vi "QTrkFree.vi"(4 "error in (no error)":errorcluster, 7 "QTrk Instance":T1={"QTrk Pointer"=0, "QTrk Settings"={"Image width"=150, "Image height"=150, "Number of threads (CPU based)"=-1, "Max Queue Size"=128, "XCOR Profile Length"=32, "XCOR Profile Width"=2, "XCOR Iterations"=5, "ZLUT MinRadius"=50.0, "ZLUT MaxRadius"=64.0, "ZLUT AngularSteps"=0, "QI Iterations"=64, "QI RadialSteps"=64, "QI AngularSteps Per Quadrant"=2, "QI MinRadius"=50.0, "QI MaxRadius"=50.0, "CUDA Device# (if using cuda)"=0, "COM Background correction factor"=2.0, "ZLUT RadialSteps"=32, "Gaussian 2D Fit Iterations"=8}}) -> (0 "error out":errorcluster)   [LabVIEW 2011]
uses:
  QTrkInstance.ctl
  QTrkSettings.ctl
  QTrkDLL.vi
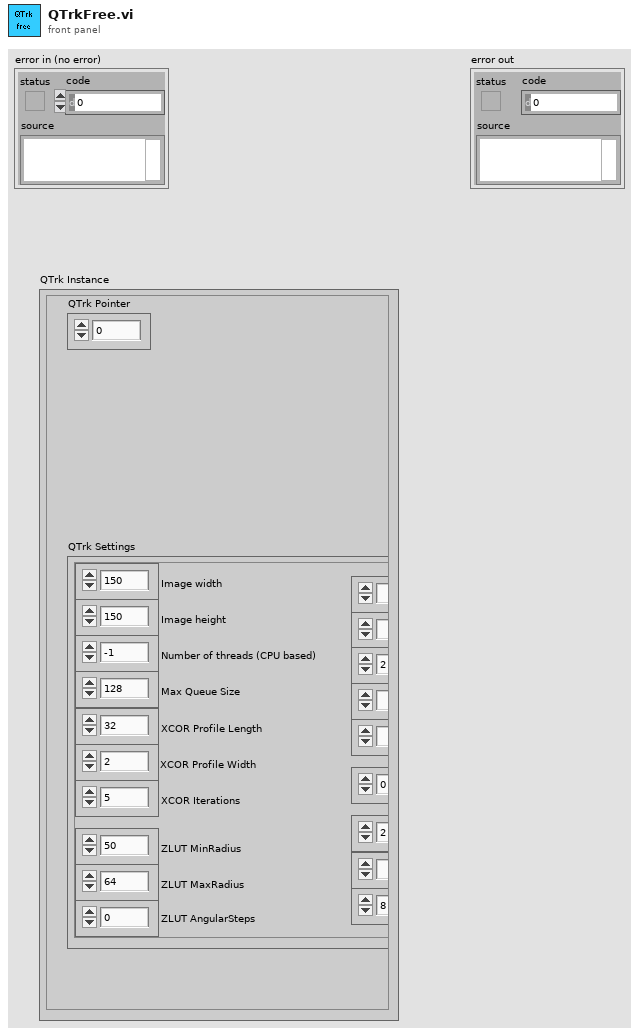
[diagram p1: front panel]
types:
  T1 = typedef "QTrkInstance.ctl" = cluster{"QTrk Pointer":u64, "QTrk Settings":T2}
  T2 = typedef "QTrkSettings.ctl" = cluster{"Image width":i32, "Image height":i32, "Number of threads (CPU based)":i32, "Max Queue Size":i32, "XCOR Profile Length":i32, "XCOR Profile Width":i32, "XCOR Iterations":i32, "ZLUT MinRadius":sgl, "ZLUT MaxRadius":sgl, "ZLUT AngularSteps":i32, "QI Iterations":i32, "QI RadialSteps":i32, "QI AngularSteps Per Quadrant":i32, "QI MinRadius":sgl, "QI MaxRadius":sgl, "CUDA Device# (if using cuda)":i32, "COM Background correction factor":sgl, "ZLUT RadialSteps":i32, "Gaussian 2D Fit Iterations":i32}
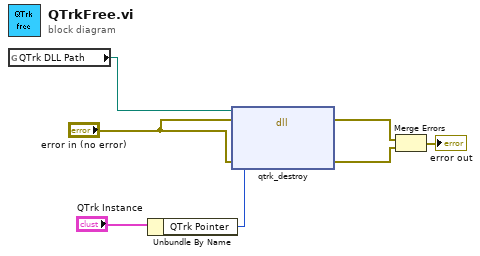
[diagram p0: block diagram]
diagram:
  n1 = global read "QTrkDLL.vi" "QTrk DLL Path"() -> (w7:path)
  n2 = Unbundle By Name("QTrk Instance") -> ("QTrk Pointer"=w5:u64)
  n3 = dll-call lib="D:/jcnossen1/cudaqi-tracker/cudatrack-labview/cputrack_d.dll" fn="qtrk_destroy"(path in=w7, error in="error in (no error)", "instance"=w5, "error"="error in (no error)") -> (error out=w3:errorcluster, "error"=w2:errorcluster)  [unwired: 3 in, 1 out]
  n4 = Merge Errors(w3, w2) -> (→"error out":errorcluster)
